vi "Reinitial Parameter After Test.vi"(8 "error in (no error)":errorcluster, 11 "main ref":T1) -> (0 "error out":errorcluster)   [LabVIEW 2025]
uses:
  controls/LAB-IQ UI Data.ctl
  Traction Loop/Traction Receipe Enum.ctl
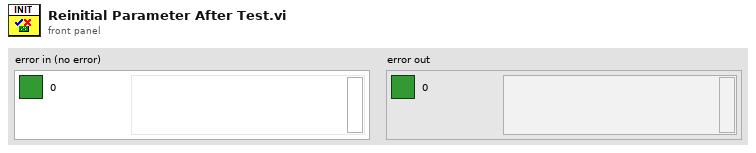
[diagram p1: front panel]
types:
  T1 = typedef "LAB-IQ UI Data.ctl" = cluster{"Main Home Screen":cluster{"GUI":refnum<vi>, "Platform Settings":refnum<vi>, "Configure":refnum<vi>, "Home":refnum<vi>, "EXIT":refnum<vi>, "service 2":refnum<vi>, "MainPage":refnum<vi>, "Analysis":refnum<vi>}, "Platform Settings":cluster{"mm/s  Surge":refnum<vi>, "Update Surge Speed":refnum<vi>, "Drive Error":refnum<vi>, "Disable Axis Jog Soft Limits":refnum<vi>, "mm/s  Sway":refnum<vi>, "Sway and Surge COM Status":refnum<vi>, "Heave COM Status":refnum<vi>, "Enable Platform":refnum<vi>, "Surge Forward Main":refnum<vi>, "Sway Right Main":refnum<vi>, "Sway Left Main":refnum<vi>, "Heave Down Main":refnum<vi>, "Heave Up main":refnum<vi>, "Update Sway Speed":refnum<vi>, "Update Heave Speed":refnum<vi>, "mm/s Heave":refnum<vi>, "mm/sec":refnum<vi>, "mm":refnum<vi>, "Surge Backward Main":refnum<vi>}, "Analysis Screen":cluster{"Analysis Home":refnum<vi>, "Surface Analysis":refnum<vi>, "Imaging":refnum<vi>, "Image Analysis":refnum<vi>, "Post Analysis":refnum<vi>}, "Config Screen":cluster{"Select Load Head":refnum<vi>, "Notes :":refnum<vi>, "FILE":refnum<vi>, "Sample ID :":refnum<vi>, "Operator ID :":refnum<vi>, "Operator Name :":refnum<vi>, "Auto":refnum<vi>}, "Motion Module":cluster{"zNL":refnum<vi>, "NL disp":refnum<vi>, "Rotary Tab":refnum<vi>, "Motion Direction:  3":refnum<vi>, "E.Velocity 2":refnum<vi>, "e.v/ssr 2":refnum<vi>, "Enter Fixed E.Velocity 2":refnum<vi>, "Enter Final SRR 2":refnum<vi>, "Enter initial SRR 2":refnum<vi>, "Enter Fixed SRR 2":refnum<vi>, "Enter the Final E.Velocity (m/s) 2":refnum<vi>, "Enter initial E.Velocity (m/s) 2":refnum<vi>, "Final Speed (RPM) 3":refnum<vi>, "Initial Speed (RPM) 2":refnum<vi>, "Enter the Final Velocity (m/s) 3":refnum<vi>, "Enter initial Velocity (m/s)  3":refnum<vi>, "Ramp Up 2":refnum<vi>, "TEST SELECTION":refnum<vi>, "SPEED SELECTION : ":refnum<vi>, "Angular Oscillation Set":refnum<vi>, "Traction":refnum<vi>, "Step Speed":refnum<vi>, "StepTable For Load-Speed":refnum<vi>, "StepTable For Speed":refnum<vi>, "Surge Forward MM":refnum<vi>, "Surge Backward MM":refnum<vi>, "M3 Image":refnum<vi>, "String 39":refnum<vi>, "Sway Left MM":refnum<vi>, "Sway Right MM":refnum<vi>, "Disable Axis Jog Soft Limits":refnum<vi>, "mm":refnum<vi>, "Heave Down MM":refnum<vi>, "Heave Up MM":refnum<vi>, "Wear Track Diameter (mm)":refnum<vi>, "Set WTD":refnum<vi>, "HomeScratch":refnum<vi>, "HomeRot":refnum<vi>, "PlaceModule":refnum<vi>, "Enter the Angle (Deg)":refnum<vi>, "Enter the Frequency (Hz)":refnum<vi>, "Motion Mode:":refnum<vi>, "LR Sway":refnum<vi>, "Rot Hor":refnum<vi>, "Scratch":refnum<vi>, "LR Cam":refnum<vi>, "MMBack":refnum<vi>, "MMNext":refnum<vi>, "Rot Ver":refnum<vi>, "Rotary Module Selection":refnum<vi>, "calculate rotary":refnum<vi>, "SPEED SELECTION : rotary":refnum<vi>, "Import 2":refnum<vi>, "Save 2":refnum<vi>, "File Path :  2":refnum<vi>, "String 45":refnum<vi>, "StepTable For Speed 3":refnum<vi>, "Enter the Speed(mm/sec)":refnum<vi>, "Enter the Speed(RPM)":refnum<vi>, "Enter Scratch Speed (mm/s):":refnum<vi>, "SwaySpeed Set":refnum<vi>, "Scartch Offset":refnum<vi>, "Motion type:":refnum<vi>, "HomeScratch 2":refnum<vi>, "Enter Scratch length (mm):":refnum<vi>, "Wear Track Diameter":refnum<vi>, "Rotary Speed Exced":refnum<vi>, "Scratch Mode":refnum<vi>, "No of Scratch":refnum<vi>}, "Environmental control":cluster{"Humidity  Status  3":refnum<vi>, "Low Temp  Status  2":refnum<vi>, "TK4 status 2":refnum<vi>, "Stage Temperature":refnum<vi>, "Sample Temperature":refnum<vi>, "Humidity (Amb)":refnum<vi>, "Clear List":refnum<vi>, "Add to list":refnum<vi>, "Wear":refnum<vi>, "Vibration":refnum<vi>, "Humidity (Chamber)":refnum<vi>, "Temperature (Chamber)":refnum<vi>, "ECR ":refnum<vi>, "Temperature (Amb)":refnum<vi>, "Microphone":refnum<vi>, "Acoustic Emission 3":refnum<vi>, "SNext":refnum<vi>, "APBack":refnum<vi>, "Enter the Temperature (°C):":refnum<vi>, "Enter the Stage \nTemperature (°C):":refnum<vi>, "Enter the Humidity (%Rh):":refnum<vi>, "Low Temp":refnum<vi>, "High Temp":refnum<vi>, "Humidity":refnum<vi>, "Sensors Picked":refnum<vi>}, "About Screen":cluster{"Password":refnum<vi>, "Home Service":refnum<vi>, "Advanced Setting":refnum<vi>, "About Tab":refnum<vi>, "ECR Port:":refnum<vi>, "Ramp Port:":refnum<vi>, "Installation/Replacement completed":refnum<vi>, "Loahead":refnum<vi>, "Heave and Surge COM Port:":refnum<vi>, "Sway COM Port:":refnum<vi>, "Temp Modbus:":refnum<vi>, "Humidity Port:":refnum<vi>, "Edit Gain Constants":refnum<vi>, "Save Gain Constants":refnum<vi>}, "Main Screen":cluster{"Main Screen Tab":refnum<vi>, "Angle and Frequency":refnum<vi>, "Stroke (mm)":refnum<vi>, "Angle (Deg)":refnum<vi>, "Main Speed Tab":refnum<vi>, "MTM MOTOR DISPLAY":refnum<vi>, "Disc Speed (m/sec)":refnum<vi>, "Ball Speed (m/sec)":refnum<vi>, "Disc Speed (RPM)":refnum<vi>, "Ball Speed (RPM)":refnum<vi>, "SPEED TAB":refnum<vi>, "Speed (m/sec)":refnum<vi>, "Set Speed (m/sec)":refnum<vi>, "Speed (RPM)":refnum<vi>, "Set Speed":refnum<vi>, "Time Tab":refnum<vi>, "Time ( HH:MM:SS ) 2":refnum<vi>, "Test Duration":refnum<vi>, "Test Duration 4":refnum<vi>, "TEST CYCLE":refnum<vi>, "TOTAL CYCLES":refnum<vi>, "Set Load (N)":refnum<vi>, "Temp Tabs":refnum<vi>, "Heater":refnum<vi>, "TK4 status":refnum<vi>, "ChamberTemp":refnum<vi>, "SetTmp":refnum<vi>, "Controller  Status":refnum<vi>, "ChamberTemp 2":refnum<vi>, "SetTmp 2":refnum<vi>, "Controller  Status 2":refnum<vi>, "ChamberTemp 3":refnum<vi>, "SetTmp 3":refnum<vi>, "Cooling":refnum<vi>, "Load Communication":refnum<vi>, "Ambient \nTemperature":refnum<vi>, "HumCOMStatus":refnum<vi>, "Ambient\n Humidity":refnum<vi>, "Freq (Hz)":refnum<vi>, "Load En":refnum<vi>, "NLt":refnum<vi>, "zNL 2":refnum<vi>, "Humidity On":refnum<vi>, "humidity disp":refnum<vi>, "Set Humidity":refnum<vi>, "NL disp 2":refnum<vi>, "Humidity On 2":refnum<vi>, "humidity disp 2":refnum<vi>, "Set Humidity 2":refnum<vi>, "NL disp 3":refnum<vi>, "AppLoadSeq scratch":refnum<vi>, "Stop Scratch":refnum<vi>, "ClrLog":refnum<vi>, "Trip Log":refnum<vi>, "STOP":refnum<vi>, "Start Test":refnum<vi>, "Test status":refnum<vi>, "AR Led":refnum<vi>, "Data":refnum<vi>, "Health":refnum<vi>, "Sway COM Status":refnum<vi>, "Heave COM Status":refnum<vi>, "Grp Tab":refnum<vi>, "Sub Graph":refnum<vi>, "SD (mm)":refnum<vi>, "Siliding distance Reset Graph":refnum<vi>, "SDGp":refnum<vi>, "Humidity Reset Graph":refnum<vi>, "HumrGp":refnum<vi>, "Acoustic Emission (mV)":refnum<vi>, "Aqucostic Reset Graph":refnum<vi>, "gACQUOS":refnum<vi>, "ECR RESET":refnum<vi>, "ECR":refnum<vi>, "Temperature Reset":refnum<vi>, "Acoustic Emission (mV) 2":refnum<vi>, "Aqucostic Reset Graph 2":refnum<vi>, "gACQUOS 2":refnum<vi>, "ECR RESET 2":refnum<vi>, "ECR 2":refnum<vi>, "Temperature Reset 2":refnum<vi>, "Temperature (deg c)":refnum<vi>, "Speed Reset Graph":refnum<vi>, "Speed Tab":refnum<vi>, "MTM DISC  SPEED":refnum<vi>, "MTM BALL SPEED":refnum<vi>, "speed mm/sec":refnum<vi>, "Hymidity":refnum<vi>, "Humidity Disable trip":refnum<vi>, "CoF Trip  2":refnum<vi>, "Depth Trip":refnum<vi>, "Weart Deapth":refnum<vi>, "Depth Reset Graph":refnum<vi>, "Weart":refnum<vi>, "Depthz":refnum<vi>, "Depth (µm)":refnum<vi>, "WearGp":refnum<vi>, "NL Trip 2":refnum<vi>, "Load pid":refnum<vi>, "Load Disable Trip":refnum<vi>, "Load Reset Graph":refnum<vi>, "NL Display 4":refnum<vi>, "Main Chart 3":refnum<vi>, "BACK":refnum<vi>, "Depth Trip 2":refnum<vi>, "COF TRIP ":refnum<vi>, "Friction Force (N)":refnum<vi>, "FF Reset Graph":refnum<vi>, "FF Disable Trip":refnum<vi>, "FF TRIP":refnum<vi>, "COF Disable Trip":refnum<vi>, "COF Reset Graph":refnum<vi>, "Start Test Temp":refnum<vi>, "zFF":refnum<vi>, "Friction Force (N) Graph":refnum<vi>, "Coefficient of Friction":refnum<vi>, "Scratch Start Test":refnum<vi>, "FF Tab":refnum<vi>, "Cyclic Friction Force (N)":refnum<vi>, "CZ FF":refnum<vi>, "Cyclic Friction Force (N) Graph":refnum<vi>, "Cyclic Coefficient of Friction":refnum<vi>, "Cyclic FF TRIP":refnum<vi>, "Cyclic FF Disable Trip":refnum<vi>, "cyclic COF Disable Trip":refnum<vi>, "cyclic COF TRIP":refnum<vi>, "cyclic COF Reset Graph":refnum<vi>, "Cyclic FF Reset Graph":refnum<vi>, "Test Trip":refnum<vi>, "Multi Scratch Pass":refnum<vi>, "Scratch Start Recording":refnum<vi>}, "Loading":cluster{"Indentation":refnum<vi>, "Reference Sample":refnum<vi>, "Load Cell Communication Slide":refnum<vi>, "com 3":refnum<vi>, "com":refnum<vi>, "DecaForce COM Status":refnum<vi>, "Update":refnum<vi>, "Clear 3":refnum<vi>, "seq":refnum<vi>, "Stribeck table":refnum<vi>, "Stribeck Table  For loading":refnum<vi>, "Loading Mode":refnum<vi>, "Enter the Final Load (N)":refnum<vi>, "Enter the CoF Trip":refnum<vi>, "Enter the Friction Force Trip":refnum<vi>, "Enter the Normal load Trip":refnum<vi>, "Enter the Load  (N)":refnum<vi>, "KiloForce":refnum<vi>, "DecaForce ":refnum<vi>, "MicroForce":refnum<vi>, "LHBack":refnum<vi>, "LHNext":refnum<vi>, "Enter the Loading Rate (N/min)":refnum<vi>, "Message":refnum<vi>, "Warning 2":refnum<vi>, "SSP 0.75":refnum<vi>, "SSP 0.5":refnum<vi>, "SSP 0.3":refnum<vi>, "Warning":refnum<vi>, "gui GIF":refnum<vi>, "Communication is established":refnum<vi>, "AppLoad 4":refnum<vi>, "Multipoint":refnum<vi>, "Load Selection":refnum<vi>}, "PID":cluster{"Ramp MulFac":refnum<vi>, "pulses LoadDiffRamp(2..10)":refnum<vi>, "PulseControlRamp(diff<=3N)":refnum<vi>, "SetLoadDeadband(%) Load(0-10N)":refnum<vi>, "PID gains out delay (microForce)":refnum<vi>, "Ramp":refnum<vi>, "Gain 2":refnum<vi>, "pulses LoadDiff(2..10)":refnum<vi>, "pulses LoadDiff(11..50)":refnum<vi>, "PulseControl(diff<=3N)":refnum<vi>, "SetLoadDeadband(%)  2":refnum<vi>, "Dummy Run":refnum<vi>, "Vertical load (N)":refnum<vi>, "AutoTune":refnum<vi>, "Offset 3 ":refnum<vi>, "apply load":refnum<vi>, "Offset  3":refnum<vi>, "apply load 2":refnum<vi>, "Enter ByPass Load":refnum<vi>, "reinit 3":refnum<vi>, "output range delay":refnum<vi>, "PID gains out delay":refnum<vi>, "Bypass Load":refnum<vi>, "pulsesSent":refnum<vi>, "pulses ":refnum<vi>, "actpid":refnum<vi>, "gFF Rot":refnum<vi>, "pulses LoadDiff(21..1000)":refnum<vi>, "Delay":refnum<vi>, "deadband":refnum<vi>}, "Config Parameters":cluster{"Tab Control 3":refnum<vi>, "Tab Control 19":refnum<vi>, "SAMPLES":refnum<vi>, "Re-initilaize":refnum<vi>, "Filter ON/OFF":refnum<vi>, "TracHomeSurgeOffsetCounts 10MM":refnum<vi>, "TracHomeSwayOffsetCounts 10MM":refnum<vi>, "Acoustic Emission:":refnum<vi>, "Apply Filter (FF)":refnum<vi>, "Filter% 2":refnum<vi>, "Apply Filter (Load)":refnum<vi>, "Filter% ":refnum<vi>, "Sway distance (mm)":refnum<vi>, "Surge distance (mm)":refnum<vi>, "DataSavingLoopDelay(ms)":refnum<vi>, "SAVE 2":refnum<vi>, "Enter Distance":refnum<vi>, "Sway Counts:":refnum<vi>, "Distance (mm): 3":refnum<vi>, "Surge Counts:":refnum<vi>, "Distance (mm): 2":refnum<vi>, "Distance (mm):":refnum<vi>, "Heave Counts:":refnum<vi>, "LRMHomeSurgeOffsetCounts":refnum<vi>, "LRMHomeSwayOffsetCounts":refnum<vi>, "TracHomeSurgeOffsetCounts 20MM":refnum<vi>, "TracHomeSwayOffsetCounts 20MM":refnum<vi>, "RotHomeSwayOffsetCounts":refnum<vi>, "RotHomeSurgeOffsetCounts":refnum<vi>, "Heave distance":refnum<vi>, "Zmm":refnum<vi>, "Heave Pulses/mm":refnum<vi>, "Surge Pulses/mm":refnum<vi>, "Sway Pulses/mm":refnum<vi>, "Heave Pitch":refnum<vi>, "Surge Pitch":refnum<vi>, "Sway Pitch":refnum<vi>, "Heave PPR":refnum<vi>, "Surge PPR":refnum<vi>, "Sway PPR":refnum<vi>, "Tab Control 5":refnum<vi>, "Tab Control 14":refnum<vi>, "Tab Control 26":refnum<vi>, "AE":refnum<vi>, "Heave Loop Delay":refnum<vi>, "Heave PID Speed":refnum<vi>, "Surge Jog Speed":refnum<vi>, "Heave Jog Speed":refnum<vi>, "Sway Loop Delay":refnum<vi>, "Sway PID Speed":refnum<vi>, "Sway Jog Speed":refnum<vi>, "DEPTH TRIP VALUE":refnum<vi>, "LOAD TRIP VALUE":refnum<vi>, "DEPTH TRIP   ENABLE":refnum<vi>, "LOAD TRIP  ENABLE":refnum<vi>, "CYCLIC FF TRIP VALUE":refnum<vi>, "FF TRIP VALUE":refnum<vi>, "CYCLIC CoF TRIP VALUE":refnum<vi>, "COF TRIP VALUE":refnum<vi>, "CYCLIC COF TRIP  ENABLE":refnum<vi>, "CYCLIC FF TRIP  ENABLE":refnum<vi>, "FF TRIP  ENABLE":refnum<vi>, "COF TRIP  ENABLE":refnum<vi>, "JOG TRIP LOAD VALUE (N)":refnum<vi>}, "Loading Com Port":cluster{"ClearAll":refnum<vi>, "Mz(Nm)":refnum<vi>, "My(Nm)":refnum<vi>, "Mx(Nm)":refnum<vi>, "Save Dwell":refnum<vi>, "Mx ":refnum<vi>, "My ":refnum<vi>, "Mz":refnum<vi>, "Fx(N)":refnum<vi>, "Fy(N)":refnum<vi>, "Fz(N)":refnum<vi>, "ZeroAll":refnum<vi>, "Acq Delay (ms)":refnum<vi>, "Burst Delay (ms)":refnum<vi>, "model":refnum<vi>, "SN":refnum<vi>, "FFx(N)":refnum<vi>, "Sensor IP":refnum<vi>, "Port":refnum<vi>, "FFy(N)":refnum<vi>, "Load(N)":refnum<vi>, "delete Handle":refnum<vi>, "Create Handle":refnum<vi>, "ft_data":refnum<vi>, "ft_range":refnum<vi>, "ft_data 2":refnum<vi>, "stop 6":refnum<vi>, "running_flag":refnum<vi>, "ft_udp_handle":refnum<vi>, "get-data-return":refnum<vi>, "get-range-return":refnum<vi>, "zero-return":refnum<vi>, "filter-return":refnum<vi>, "initial-return":refnum<vi>, "deleteHandle-result":refnum<vi>, "Load Cell Temp":refnum<vi>}, "Heave AND Surge":cluster{"SURGE POSE":refnum<vi>, "error out Read":refnum<vi>, "HEAVE POSE":refnum<vi>, "State":refnum<vi>, "Homed":refnum<vi>, "Sequence ID":refnum<vi>, "error out Write":refnum<vi>, "faultCode":refnum<vi>, "Ack ID":refnum<vi>, "SPEED":refnum<vi>, "Distance":refnum<vi>, "Mode Command":refnum<vi>, "Heave and Surge Read":refnum<vi>, "Read Heave Temp":refnum<vi>, "Spare 15":refnum<vi>, "Spare 14":refnum<vi>, "Spare 13":refnum<vi>, "Spare 12":refnum<vi>, "Spare 11":refnum<vi>, "Spare 10":refnum<vi>, "Spare 9":refnum<vi>, "Spare 8":refnum<vi>, "Spare 7":refnum<vi>, "Spare 6":refnum<vi>, "Spare 5":refnum<vi>, "Spare 4":refnum<vi>, "Spare 2":refnum<vi>, "Spare 1":refnum<vi>, "Node Id":refnum<vi>, "Spare 3":refnum<vi>, "SPARE 4":refnum<vi>, "SPARE 3":refnum<vi>, "SPARE 2":refnum<vi>, "SPARE 1":refnum<vi>, "fwMajor":refnum<vi>, "fwMinor":refnum<vi>, "Manual Write":refnum<vi>, "Heave and Surge Write":refnum<vi>, "SPARE 5":refnum<vi>, "Reserved ":refnum<vi>, "SPARE 8":refnum<vi>, "SPARE 6":refnum<vi>, "SPARE 7":refnum<vi>, "SPARE 17":refnum<vi>, "SPARE 16":refnum<vi>, "SPARE 15":refnum<vi>, "SPARE 14":refnum<vi>, "SPARE 13":refnum<vi>, "SPARE 12":refnum<vi>, "SPARE 11":refnum<vi>, "SPARE 10":refnum<vi>, "SPARE 9":refnum<vi>, "System UPTIME":refnum<vi>, "Missed Packets":refnum<vi>, "faultCode Surge Right":refnum<vi>, "faultCode Surge Left":refnum<vi>, "faultCode Heave":refnum<vi>, "UPLINK HEAVE":refnum<vi>, "DOWNLINK HEAVE":refnum<vi>}, "New PID LOGIC":cluster{"Fine Tune Zone":refnum<vi>, "PID SDelay":refnum<vi>, "Max_pos_limit":refnum<vi>, "Min_pos_limit":refnum<vi>, "i_limit":refnum<vi>, "pct_scale":refnum<vi>, "Deadband":refnum<vi>, "Kd":refnum<vi>, "Ki":refnum<vi>, "Kp":refnum<vi>, "Current Position":refnum<vi>, "Set Load":refnum<vi>, "Current Load":refnum<vi>, "Pulse delta":refnum<vi>, "Init Step":refnum<vi>, "Max Step Linit":refnum<vi>, "min_deadband_floor":refnum<vi>, "dynamic_spindle_noise_scalar":refnum<vi>, "min_finetune_floor":refnum<vi>, "filter_alpha":refnum<vi>}, "SWAY ":cluster{"fwMajor":refnum<vi>, "Homed":refnum<vi>, "Rotary POSE":refnum<vi>, "State":refnum<vi>, "SWAY POSE":refnum<vi>, "Ack ID":refnum<vi>, "faultCode":refnum<vi>, "Node Id":refnum<vi>, "fwMinor":refnum<vi>, "Spare 6":refnum<vi>, "Spare 5":refnum<vi>, "Spare 4":refnum<vi>, "Spare 3":refnum<vi>, "Spare 2":refnum<vi>, "Spare 1":refnum<vi>, "Spare 7":refnum<vi>, "SPARE  5":refnum<vi>, "error out Write  SWAY ":refnum<vi>, "error out Read SWAY ":refnum<vi>, "Manual Write SWAY ":refnum<vi>, "SWAY WRITE":refnum<vi>, "SPARE  4":refnum<vi>, "SPARE  3":refnum<vi>, "SPARE 2":refnum<vi>, "SPARE 1":refnum<vi>, "Spare 15":refnum<vi>, "Spare 14":refnum<vi>, "Spare 13":refnum<vi>, "Spare 12":refnum<vi>, "Spare 11":refnum<vi>, "Spare 9":refnum<vi>, "Spare 8":refnum<vi>, "SPEED":refnum<vi>, "Distance":refnum<vi>, "Mode Command":refnum<vi>, "Sequence ID":refnum<vi>, "SWAY READ":refnum<vi>, "Spare 10":refnum<vi>, "Read SWAY Temp":refnum<vi>, "faultCode Sway ":refnum<vi>, "Missed Packets":refnum<vi>, "System UPTIME sway":refnum<vi>, "SPARE 6":refnum<vi>, "SPARE 7":refnum<vi>, "SPARE 9":refnum<vi>, "SPARE 11":refnum<vi>, "SPARE 10":refnum<vi>, "SPARE 8":refnum<vi>, "SPARE 13":refnum<vi>, "SPARE 12":refnum<vi>, "SPARE 17":refnum<vi>, "SPARE 16":refnum<vi>, "SPARE 15":refnum<vi>, "SPARE 14":refnum<vi>, "Reserved":refnum<vi>, "faultCode Rotary":refnum<vi>, "UPLINK SWAY":refnum<vi>, "DOWNLINK SWAY":refnum<vi>}, "Analysis Screen":cluster{"Analysis Home":refnum<vi>, "Refresh 2":refnum<vi>, "MEAN 4":refnum<vi>, "SD 4":refnum<vi>, "VARIANCE 4":refnum<vi>, "MEAN  3":refnum<vi>, "SD  3":refnum<vi>, "VARIANCE  3":refnum<vi>, "MEAN 2":refnum<vi>, "SD  2":refnum<vi>, "VARIANCE 2":refnum<vi>, "MEAN":refnum<vi>, "SD":refnum<vi>, "VARIANCE":refnum<vi>, "File 4 Discription":refnum<vi>, "OPEN 4":refnum<vi>, "File Name 4":refnum<vi>, "OPEN 3":refnum<vi>, "File 3 Discription":refnum<vi>, "File Name 3":refnum<vi>, "Y-AXIS":refnum<vi>, "X-AXIS":refnum<vi>, "XY Graph":refnum<vi>, "File Name 2":refnum<vi>, "File Name 1":refnum<vi>, "OPEN 2":refnum<vi>, "OPEN 1":refnum<vi>, "File 1 Discription ":refnum<vi>, "File 2 Discription":refnum<vi>, "Export":refnum<vi>, "File Format":refnum<vi>}, "Traction":cluster{"faultCode Traction 2":refnum<vi>, "faultCode Traction 1":refnum<vi>, "Missed Packets":refnum<vi>, "System UPTIME Traction":refnum<vi>, "SPARE 17":refnum<vi>, "SPARE 16":refnum<vi>, "SPARE 15":refnum<vi>, "SPARE 14":refnum<vi>, "SPARE 13":refnum<vi>, "SPARE 12":refnum<vi>, "SPARE 11":refnum<vi>, "SPARE 10":refnum<vi>, "SPARE 9":refnum<vi>, "SPARE 8":refnum<vi>, "SPARE 7":refnum<vi>, "SPARE 6":refnum<vi>, "Reserved":refnum<vi>, "SPARE  5":refnum<vi>, "Manual Write TRACTION":refnum<vi>, "TRACTION WRITE":refnum<vi>, "SPARE  4":refnum<vi>, "SPARE  3":refnum<vi>, "SPARE 2":refnum<vi>, "SPARE 1":refnum<vi>, "Spare 7":refnum<vi>, "Spare 6":refnum<vi>, "Spare 5":refnum<vi>, "Spare 4":refnum<vi>, "Spare 2":refnum<vi>, "Spare 1":refnum<vi>, "Node Id":refnum<vi>, "Read TRACTION Temp":refnum<vi>, "fwMinor":refnum<vi>, "fwMajor":refnum<vi>, "faultCode":refnum<vi>, "TRACTION POSE":refnum<vi>, "TRACTION POSE 2":refnum<vi>, "Homed":refnum<vi>, "State":refnum<vi>, "Ack ID":refnum<vi>, "SPEED":refnum<vi>, "Distance":refnum<vi>, "Mode Command":refnum<vi>, "Sequence ID":refnum<vi>, "error out Read TRACTION":refnum<vi>, "error out Write  TRACTION":refnum<vi>, "TRACTION READ":refnum<vi>, "Spare 3":refnum<vi>}, "Traction reciepe":cluster{"SRR Sweep Range (%) Stribeck":refnum<vi>, "Traction Receipe":refnum<vi>, "Total Execution Time":refnum<vi>, "Total Steps":refnum<vi>, "Duration / Step (s)  Stribeck":refnum<vi>, "STRIBECK Fixed SRR List (%)":refnum<vi>, "Duration / Step (s) Traction":refnum<vi>, "SRR Sweep Range (%) traction":refnum<vi>, "Rolling Speed (mm/s)":refnum<vi>, "Temperature Stages (°C)":refnum<vi>, "Ball Load (N)":refnum<vi>, "Lubricant Name":refnum<vi>, "Profile File Name":refnum<vi>, "SET entrainment Velocity":refnum<vi>, "Test Array Size":refnum<vi>, "SRR INDEX [ STRIBECK]":refnum<vi>, "Stribeck Size":refnum<vi>, "SET SRR":refnum<vi>, "ELAPSED TIMER ":refnum<vi>, "BALL SET RPM":refnum<vi>, "DISC SET RPM":refnum<vi>, "SET LOAD":refnum<vi>, "TEMPERATURE READ":refnum<vi>, "SET TEMPERATURE":refnum<vi>, "Traction Size":refnum<vi>, "DISC SPEED (rpm)":refnum<vi>, "BALL SPEED (rpm)":refnum<vi>, "BALL WEAR TRACK":refnum<vi>, "DISC WEARTRACK":refnum<vi>, "SRR INDEX [ TRACTION]":refnum<vi>, "Start Index Type":refnum<vi>, "Enum - Menu":refnum<vi>, "Ball (mm/sec)":refnum<vi>, "Disc (mm/sec)":refnum<vi>}, "Traction Control":cluster{"HomeTraction":refnum<vi>, "Demo Mode Display":refnum<vi>, "Traction Message":refnum<vi>, "Traction Step Update Details":refnum<vi>, "Main Tab sequence for selection":refnum<vi>, "Ramp Tab":refnum<vi>, "e.v/ssr":refnum<vi>, "Enter Fixed E.Velocity":refnum<vi>, "Enter Final SRR":refnum<vi>, "Enter initial SRR":refnum<vi>, "Enter Fixed SRR":refnum<vi>, "Enter the Final E.Velocity (m/s)":refnum<vi>, "Enter initial E.Velocity (m/s)":refnum<vi>, "Ball WTD":refnum<vi>, "E.Velocity":refnum<vi>, "Enter the Final Velocity (m/s)":refnum<vi>, "Enter initial Velocity (m/s)":refnum<vi>, "Ramp Up   Disc":refnum<vi>, "Initial DiscSpeed (RPM)":refnum<vi>, "Final Speed (RPM) Ball":refnum<vi>, "Final Speed (RPM)":refnum<vi>, "Initial Speed (RPM) Ball":refnum<vi>, "Enter the Final Velocity (m/s) Ball":refnum<vi>, "Enter initial Velocity (m/s) Ball":refnum<vi>, "Ramp Up":refnum<vi>, "ExceedBallSpeed step":refnum<vi>, "ExceedDiscSpeed":refnum<vi>, "BallSpeed Exceed Indication":refnum<vi>, "Apply":refnum<vi>, "SPEED SELECTION : MTM":refnum<vi>, "SPEED SELECTION : MTM 2":refnum<vi>, "TEST SELECTION (MTM)":refnum<vi>, "MTM Test Selection":refnum<vi>, "File Path Tab":refnum<vi>, "File Path String":refnum<vi>, "Save":refnum<vi>, "Save  2":refnum<vi>, "Import ":refnum<vi>, "File Path :":refnum<vi>, "Step Sequence Indication Tab":refnum<vi>, "Step Sequence Indication":refnum<vi>, "Calculate Step":refnum<vi>, "StepTable":refnum<vi>, "ExceedDiscSpeed  Cinstant Speed":refnum<vi>, "ExceedBallSpeed Constant":refnum<vi>, "TEST SELECTION (MTM) 2":refnum<vi>, "SPEED SELECTION : MTM 3":refnum<vi>, "MTM Test Selection 2":refnum<vi>, "Enter the Speed (m/sec): ":refnum<vi>, "Enter the Speed (m/sec):  2":refnum<vi>, "Enter the Speed (RPM):":refnum<vi>, "Lower Spped ":refnum<vi>, "Upper":refnum<vi>, "Enter the Speed (RPM):Ball":refnum<vi>, "Disc Motion Direction: ":refnum<vi>, "Ball Motion Direction :":refnum<vi>, "Motion Mode: ":refnum<vi>, "Wear Track Diameter (mm) ":refnum<vi>, "Disc Speed Indicator":refnum<vi>, "ExceedBallSpeed":refnum<vi>}, "Acquostic":cluster{"Last Config Rejected ":refnum<vi>, "rx command count":refnum<vi>, "Current Filter Id":refnum<vi>, "Isolated Gain":refnum<vi>, "DAQ Status":refnum<vi>, "error out":refnum<vi>, "error in (no error)":refnum<vi>, "Uplink Packet":refnum<vi>, "data out":refnum<vi>, "Downlink Packet":refnum<vi>, "Signal Energy":refnum<vi>, "Amplitude db_AE":refnum<vi>, "Peak Amplitude":refnum<vi>, "AE Ring-Down Counts":refnum<vi>, "Gains":refnum<vi>, "Manual Write Acquostic":refnum<vi>}}
  T2 = enum8{"Enabled", "Disabled", "Disabled and Grayed Out"}
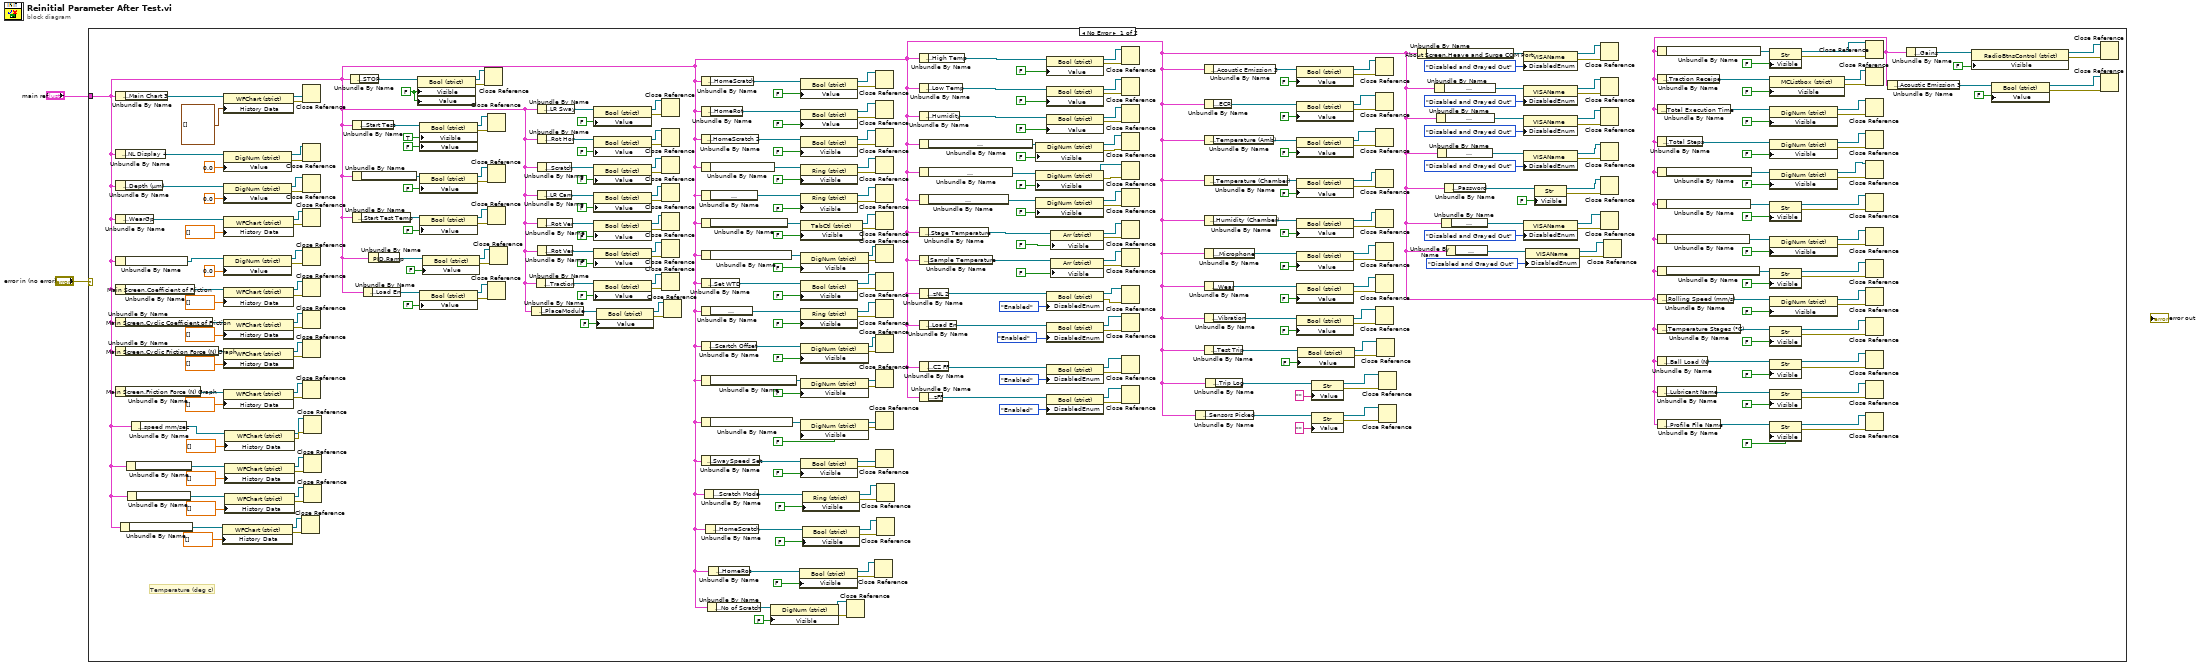
[diagram p0: block diagram]
diagram:
  n1 = case shown="No Error" "error in (no error)" {
    tunnel: "main ref" -> [w4 _]
    frame No Error {
      w293 = FALSE ("Visible")
      # "Temperature (deg c)"
      n2 = Unbundle By Name(w4) -> ("Main Screen.Main Chart 3"=w358:refnum<vi>)
      n3 = Unbundle By Name(w4) -> ("Main Screen.NL Display 4"=w356:refnum<vi>)
      n4 = Unbundle By Name(w4) -> ("Main Screen.Depth (µm)"=w351:refnum<vi>)
      n5 = Unbundle By Name(w4) -> ("Main Screen.WearGp"=w348:refnum<vi>)
      n6 = Unbundle By Name(w4) -> ("Main Screen.Time ( HH:MM:SS ) 2"=w344:refnum<vi>)
      n7 = Unbundle By Name(w4) -> ("Main Screen.Coefficient of Friction"=w341:refnum<vi>)
      n8 = Unbundle By Name(w4) -> ("Main Screen.Cyclic Coefficient of Friction"=w333:refnum<vi>)
      n9 = Unbundle By Name(w4) -> ("Main Screen.Cyclic Friction Force (N) Graph"=w337:refnum<vi>)
      n10 = Unbundle By Name(w4) -> ("Main Screen.Friction Force (N) Graph"=w329:refnum<vi>)
      n11 = Unbundle By Name(w4) -> ("Main Screen.Temperature (deg c)"=w312:refnum<vi>)
      n12 = Unbundle By Name(w4) -> ("Main Screen.MTM DISC  SPEED"=w319:refnum<vi>)
      n13 = Unbundle By Name(w4) -> ("Main Screen.MTM BALL SPEED"=w314:refnum<vi>)
      n14 = Unbundle By Name(w4) -> ("Main Screen.speed mm/sec"=w322:refnum<vi>)
      n15 = property class="WFChart (strict)"(reference=w312, "History Data"=dbl[] []) -> (reference out=w309:refnum<vi>, error out=w311:errorcluster)  [unwired: 1 in]
      n16 = property class="WFChart (strict)"(reference=w358, "History Data"=cluster{dbl, "NL disp":dbl, dbl}[] []) -> (reference out=w360:refnum<vi>, error out=w359:errorcluster)  [unwired: 1 in]
      n17 = property class="DigNum (strict)"(reference=w356, "Value"=0.0) -> (reference out=w354:refnum<vi>, error out=w355:errorcluster)  [unwired: 1 in]
      n18 = property class="DigNum (strict)"(reference=w351, "Value"=0.0) -> (reference out=w352:refnum<vi>, error out=w350:errorcluster)  [unwired: 1 in]
      n19 = property class="WFChart (strict)"(reference=w348, "History Data"=dbl[] []) -> (reference out=w346:refnum<vi>, error out=w347:errorcluster)  [unwired: 1 in]
      n20 = property class="DigNum (strict)"(reference=w344, "Value"=0.0) -> (reference out=w325:refnum<vi>, error out=w345:errorcluster)  [unwired: 1 in]
      n21 = property class="WFChart (strict)"(reference=w341, "History Data"=dbl[] []) -> (reference out=w342:refnum<vi>, error out=w340:errorcluster)  [unwired: 1 in]
      n22 = property class="WFChart (strict)"(reference=w333, "History Data"=dbl[] []) -> (reference out=w332:refnum<vi>, error out=w334:errorcluster)  [unwired: 1 in]
      n23 = property class="WFChart (strict)"(reference=w337, "History Data"=dbl[] []) -> (reference out=w335:refnum<vi>, error out=w336:errorcluster)  [unwired: 1 in]
      n24 = property class="WFChart (strict)"(reference=w329, "History Data"=dbl[] []) -> (reference out=w327:refnum<vi>, error out=w328:errorcluster)  [unwired: 1 in]
      n25 = property class="WFChart (strict)"(reference=w322, "History Data"=dbl[] []) -> (reference out=w321:refnum<vi>, error out=w323:errorcluster)  [unwired: 1 in]
      n26 = property class="WFChart (strict)"(reference=w319, "History Data"=dbl[] []) -> (reference out=w320:refnum<vi>, error out=w318:errorcluster)  [unwired: 1 in]
      n27 = property class="WFChart (strict)"(reference=w314, "History Data"=dbl[] []) -> (reference out=w313:refnum<vi>, error out=w315:errorcluster)  [unwired: 1 in]
      n28 = Close Reference(reference=w309, error in (no error)=w311) -> ()  [unwired: 1 out]
      n29 = Close Reference(reference=w360, error in (no error)=w359) -> ()  [unwired: 1 out]
      n30 = Close Reference(reference=w354, error in (no error)=w355) -> ()  [unwired: 1 out]
      n31 = Close Reference(reference=w352, error in (no error)=w350) -> ()  [unwired: 1 out]
      n32 = Close Reference(reference=w346, error in (no error)=w347) -> ()  [unwired: 1 out]
      n33 = Close Reference(reference=w325, error in (no error)=w345) -> ()  [unwired: 1 out]
      n34 = Close Reference(reference=w342, error in (no error)=w340) -> ()  [unwired: 1 out]
      n35 = Close Reference(reference=w332, error in (no error)=w334) -> ()  [unwired: 1 out]
      n36 = Close Reference(reference=w335, error in (no error)=w336) -> ()  [unwired: 1 out]
      n37 = Close Reference(reference=w327, error in (no error)=w328) -> ()  [unwired: 1 out]
      n38 = Close Reference(reference=w321, error in (no error)=w323) -> ()  [unwired: 1 out]
      n39 = Close Reference(reference=w320, error in (no error)=w318) -> ()  [unwired: 1 out]
      n40 = Close Reference(reference=w313, error in (no error)=w315) -> ()  [unwired: 1 out]
      n41 = Unbundle By Name(w4) -> ("Main Screen.STOP"=w299:refnum<vi>)
      n42 = Unbundle By Name(w4) -> ("Main Screen.Start Test"=w297:refnum<vi>)
      n43 = Unbundle By Name(w4) -> ("Main Screen.Scratch Start Test"=w305:refnum<vi>)
      n44 = Unbundle By Name(w4) -> ("Main Screen.Start Test Temp"=w306:refnum<vi>)
      n45 = Unbundle By Name(w4) -> ("Main Screen.Load En"=w285:refnum<vi>)
      n46 = Unbundle By Name(w4) -> ("PID.Ramp"=w290:refnum<vi>)
      n47 = property class="Bool (strict)"(reference=w299, "Visible"=w293, "Value"=w293) -> (reference out=w294:refnum<vi>, error out=w300:errorcluster)  [unwired: 1 in]
      n48 = property class="Bool (strict)"(reference=w297, "Visible"=TRUE, "Value"=FALSE) -> (reference out=w295:refnum<vi>, error out=w296:errorcluster)  [unwired: 1 in]
      n49 = property class="Bool (strict)"(reference=w305, "Value"=FALSE) -> (reference out=w303:refnum<vi>, error out=w304:errorcluster)  [unwired: 1 in]
      n50 = property class="Bool (strict)"(reference=w306, "Value"=FALSE) -> (reference out=w308:refnum<vi>, error out=w307:errorcluster)  [unwired: 1 in]
      n51 = property class="Bool (strict)"(reference=w285, "Value"=FALSE) -> (reference out=w287:refnum<vi>, error out=w286:errorcluster)  [unwired: 1 in]
      n52 = property class="Bool (strict)"(reference=w290, "Value"=FALSE) -> (reference out=w288:refnum<vi>, error out=w289:errorcluster)  [unwired: 1 in]
      n53 = Close Reference(reference=w294, error in (no error)=w300) -> ()  [unwired: 1 out]
      n54 = Close Reference(reference=w295, error in (no error)=w296) -> ()  [unwired: 1 out]
      n55 = Close Reference(reference=w303, error in (no error)=w304) -> ()  [unwired: 1 out]
      n56 = Close Reference(reference=w308, error in (no error)=w307) -> ()  [unwired: 1 out]
      n57 = Close Reference(reference=w287, error in (no error)=w286) -> ()  [unwired: 1 out]
      n58 = Close Reference(reference=w288, error in (no error)=w289) -> ()  [unwired: 1 out]
      n59 = Unbundle By Name(w4) -> ("Motion Module.PlaceModule"=w254:refnum<vi>)
      n60 = Unbundle By Name(w4) -> ("Motion Module.Traction"=w258:refnum<vi>)
      n61 = Unbundle By Name(w4) -> ("Motion Module.LR Sway"=w281:refnum<vi>)
      n62 = Unbundle By Name(w4) -> ("Motion Module.Rot Hor"=w278:refnum<vi>)
      n63 = Unbundle By Name(w4) -> ("Motion Module.Scratch"=w274:refnum<vi>)
      n64 = Unbundle By Name(w4) -> ("Motion Module.LR Cam"=w269:refnum<vi>)
      n65 = Unbundle By Name(w4) -> ("Motion Module.Rot Ver"=w266:refnum<vi>)
      n66 = Unbundle By Name(w4) -> ("Motion Module.Rot Ver"=w262:refnum<vi>)
      n67 = property class="Bool (strict)"(reference=w281, "Value"=FALSE) -> (reference out=w283:refnum<vi>, error out=w282:errorcluster)  [unwired: 1 in]
      n68 = property class="Bool (strict)"(reference=w278, "Value"=FALSE) -> (reference out=w276:refnum<vi>, error out=w277:errorcluster)  [unwired: 1 in]
      n69 = property class="Bool (strict)"(reference=w274, "Value"=FALSE) -> (reference out=w272:refnum<vi>, error out=w275:errorcluster)  [unwired: 1 in]
      n70 = property class="Bool (strict)"(reference=w269, "Value"=FALSE) -> (reference out=w271:refnum<vi>, error out=w268:errorcluster)  [unwired: 1 in]
      n71 = property class="Bool (strict)"(reference=w266, "Value"=FALSE) -> (reference out=w264:refnum<vi>, error out=w267:errorcluster)  [unwired: 1 in]
      n72 = property class="Bool (strict)"(reference=w262, "Value"=FALSE) -> (reference out=w260:refnum<vi>, error out=w261:errorcluster)  [unwired: 1 in]
      n73 = property class="Bool (strict)"(reference=w258, "Value"=FALSE) -> (reference out=w256:refnum<vi>, error out=w257:errorcluster)  [unwired: 1 in]
      n74 = property class="Bool (strict)"(reference=w254, "Value"=FALSE) -> (reference out=w252:refnum<vi>, error out=w253:errorcluster)  [unwired: 1 in]
      n75 = Close Reference(reference=w283, error in (no error)=w282) -> ()  [unwired: 1 out]
      n76 = Close Reference(reference=w276, error in (no error)=w277) -> ()  [unwired: 1 out]
      n77 = Close Reference(reference=w272, error in (no error)=w275) -> ()  [unwired: 1 out]
      n78 = Close Reference(reference=w271, error in (no error)=w268) -> ()  [unwired: 1 out]
      n79 = Close Reference(reference=w264, error in (no error)=w267) -> ()  [unwired: 1 out]
      n80 = Close Reference(reference=w260, error in (no error)=w261) -> ()  [unwired: 1 out]
      n81 = Close Reference(reference=w256, error in (no error)=w257) -> ()  [unwired: 1 out]
      n82 = Close Reference(reference=w252, error in (no error)=w253) -> ()  [unwired: 1 out]
      n83 = Unbundle By Name(w4) -> ("Motion Module.HomeScratch"=w222:refnum<vi>)
      n84 = Unbundle By Name(w4) -> ("Motion Module.HomeRot"=w225:refnum<vi>)
      n85 = Unbundle By Name(w4) -> ("Motion Module.HomeScratch 2"=w229:refnum<vi>)
      n86 = Unbundle By Name(w4) -> ("Motion Module.Motion Direction:  3"=w234:refnum<vi>)
      n87 = Unbundle By Name(w4) -> ("Motion Module.Motion Mode:"=w237:refnum<vi>)
      n88 = Unbundle By Name(w4) -> ("Motion Module.Rotary Module Selection"=w241:refnum<vi>)
      n89 = Unbundle By Name(w4) -> ("Motion Module.Wear Track Diameter (mm)"=w245:refnum<vi>)
      n90 = Unbundle By Name(w4) -> ("Motion Module.Set WTD"=w249:refnum<vi>)
      n91 = Unbundle By Name(w4) -> ("Motion Module.Motion type:"=w218:refnum<vi>)
      n92 = Unbundle By Name(w4) -> ("Motion Module.Scartch Offset"=w215:refnum<vi>)
      n93 = Unbundle By Name(w4) -> ("Motion Module.Enter Scratch Speed (mm/s):"=w210:refnum<vi>)
      n94 = Unbundle By Name(w4) -> ("Motion Module.Enter Scratch length (mm):"=w206:refnum<vi>)
      n95 = Unbundle By Name(w4) -> ("Motion Module.SwaySpeed Set"=w202:refnum<vi>)
      n96 = Unbundle By Name(w4) -> ("Motion Module.Scratch Mode"=w151:refnum<vi>)
      n97 = Unbundle By Name(w4) -> ("Motion Module.HomeScratch"=w146:refnum<vi>)
      n98 = Unbundle By Name(w4) -> ("Motion Module.No of Scratch"=w66:refnum<vi>)
      n99 = Unbundle By Name(w4) -> ("Motion Module.HomeRot"=w143:refnum<vi>)
      n100 = property class="DigNum (strict)"(reference=w66, "Visible"=FALSE) -> (reference out=w67:refnum<vi>, error out=w65:errorcluster)  [unwired: 1 in]
      n101 = property class="Bool (strict)"(reference=w143, "Visible"=FALSE ("Value")) -> (reference out=w141:refnum<vi>, error out=w144:errorcluster)  [unwired: 1 in]
      n102 = property class="Bool (strict)"(reference=w222, "Value"=FALSE) -> (reference out=w220:refnum<vi>, error out=w221:errorcluster)  [unwired: 1 in]
      n103 = property class="Bool (strict)"(reference=w225, "Value"=FALSE) -> (reference out=w227:refnum<vi>, error out=w226:errorcluster)  [unwired: 1 in]
      n104 = property class="Bool (strict)"(reference=w229, "Visible"=FALSE ("Value")) -> (reference out=w231:refnum<vi>, error out=w228:errorcluster)  [unwired: 1 in]
      n105 = property class="Ring (strict)"(reference=w234, "Visible"=FALSE ("Value")) -> (reference out=w232:refnum<vi>, error out=w235:errorcluster)  [unwired: 1 in]
      n106 = property class="Ring (strict)"(reference=w237, "Visible"=FALSE ("Value")) -> (reference out=w239:refnum<vi>, error out=w236:errorcluster)  [unwired: 1 in]
      n107 = property class="TabCtl (strict)"(reference=w241, "Visible"=FALSE ("Value")) -> (reference out=w243:refnum<vi>, error out=w242:errorcluster)  [unwired: 1 in]
      n108 = property class="DigNum (strict)"(reference=w245, "Visible"=FALSE ("Value")) -> (reference out=w247:refnum<vi>, error out=w246:errorcluster)  [unwired: 1 in]
      n109 = property class="Bool (strict)"(reference=w249, "Visible"=FALSE ("Value")) -> (reference out=w251:refnum<vi>, error out=w250:errorcluster)  [unwired: 1 in]
      n110 = property class="Ring (strict)"(reference=w218, "Visible"=FALSE ("Value")) -> (reference out=w213:refnum<vi>, error out=w217:errorcluster)  [unwired: 1 in]
      n111 = property class="DigNum (strict)"(reference=w215, "Visible"=FALSE ("Value")) -> (reference out=w212:refnum<vi>, error out=w214:errorcluster)  [unwired: 1 in]
      n112 = property class="DigNum (strict)"(reference=w210, "Visible"=FALSE ("Value")) -> (reference out=w208:refnum<vi>, error out=w209:errorcluster)  [unwired: 1 in]
      n113 = property class="DigNum (strict)"(reference=w206, "Visible"=FALSE ("Value")) -> (reference out=w204:refnum<vi>, error out=w205:errorcluster)  [unwired: 1 in]
      n114 = property class="Bool (strict)"(reference=w202, "Visible"=FALSE ("Value")) -> (reference out=w200:refnum<vi>, error out=w201:errorcluster)  [unwired: 1 in]
      n115 = property class="Ring (strict)"(reference=w151, "Visible"=FALSE ("Value")) -> (reference out=w149:refnum<vi>, error out=w152:errorcluster)  [unwired: 1 in]
      n116 = property class="Bool (strict)"(reference=w146, "Visible"=FALSE ("Value")) -> (reference out=w148:refnum<vi>, error out=w145:errorcluster)  [unwired: 1 in]
      n117 = Close Reference(reference=w67, error in (no error)=w65) -> ()  [unwired: 1 out]
      n118 = Close Reference(reference=w141, error in (no error)=w144) -> ()  [unwired: 1 out]
      n119 = Close Reference(reference=w220, error in (no error)=w221) -> ()  [unwired: 1 out]
      n120 = Close Reference(reference=w227, error in (no error)=w226) -> ()  [unwired: 1 out]
      n121 = Close Reference(reference=w231, error in (no error)=w228) -> ()  [unwired: 1 out]
      n122 = Close Reference(reference=w232, error in (no error)=w235) -> ()  [unwired: 1 out]
      n123 = Close Reference(reference=w239, error in (no error)=w236) -> ()  [unwired: 1 out]
      n124 = Close Reference(reference=w243, error in (no error)=w242) -> ()  [unwired: 1 out]
      n125 = Close Reference(reference=w247, error in (no error)=w246) -> ()  [unwired: 1 out]
      n126 = Close Reference(reference=w251, error in (no error)=w250) -> ()  [unwired: 1 out]
      n127 = Close Reference(reference=w213, error in (no error)=w217) -> ()  [unwired: 1 out]
      n128 = Close Reference(reference=w212, error in (no error)=w214) -> ()  [unwired: 1 out]
      n129 = Close Reference(reference=w208, error in (no error)=w209) -> ()  [unwired: 1 out]
      n130 = Close Reference(reference=w204, error in (no error)=w205) -> ()  [unwired: 1 out]
      n131 = Close Reference(reference=w200, error in (no error)=w201) -> ()  [unwired: 1 out]
      n132 = Close Reference(reference=w149, error in (no error)=w152) -> ()  [unwired: 1 out]
      n133 = Close Reference(reference=w148, error in (no error)=w145) -> ()  [unwired: 1 out]
      n134 = Unbundle By Name(w4) -> ("Environmental control.High Temp"=w170:refnum<vi>)
      n135 = Unbundle By Name(w4) -> ("Environmental control.Low Temp"=w173:refnum<vi>)
      n136 = Unbundle By Name(w4) -> ("Environmental control.Humidity"=w177:refnum<vi>)
      n137 = Unbundle By Name(w4) -> ("Environmental control.Enter the Stage \nTemperature (°C):"=w182:refnum<vi>)
      n138 = Unbundle By Name(w4) -> ("Environmental control.Enter the Temperature (°C):"=w185:refnum<vi>)
      n139 = Unbundle By Name(w4) -> ("Environmental control.Enter the Humidity (%Rh):"=w189:refnum<vi>)
      n140 = Unbundle By Name(w4) -> ("Environmental control.Stage Temperature"=w193:refnum<vi>)
      n141 = Unbundle By Name(w4) -> ("Environmental control.Sample Temperature"=w197:refnum<vi>)
      n142 = Unbundle By Name(w4) -> ("Main Screen.zNL 2"=w168:refnum<vi>)
      n143 = Unbundle By Name(w4) -> ("Main Screen.Load En"=w164:refnum<vi>)
      n144 = Unbundle By Name(w4) -> ("Main Screen.CZ FF"=w158:refnum<vi>)
      n145 = Unbundle By Name(w4) -> ("Main Screen.zFF"=w155:refnum<vi>)
      n146 = property class="DigNum (strict)"(reference=w182, "Visible"=FALSE ("Value")) -> (reference out=w180:refnum<vi>, error out=w183:errorcluster)  [unwired: 1 in]
      n147 = property class="DigNum (strict)"(reference=w185, "Visible"=FALSE ("Value")) -> (reference out=w187:refnum<vi>, error out=w184:errorcluster)  [unwired: 1 in]
      n148 = property class="DigNum (strict)"(reference=w189, "Visible"=FALSE ("Value")) -> (reference out=w191:refnum<vi>, error out=w190:errorcluster)  [unwired: 1 in]
      n149 = property class="Bool (strict)"(reference=w170, "Value"=FALSE) -> (reference out=w140:refnum<vi>, error out=w169:errorcluster)  [unwired: 1 in]
      n150 = property class="Bool (strict)"(reference=w173, "Value"=FALSE) -> (reference out=w175:refnum<vi>, error out=w174:errorcluster)  [unwired: 1 in]
      n151 = property class="Bool (strict)"(reference=w177, "Value"=FALSE) -> (reference out=w179:refnum<vi>, error out=w176:errorcluster)  [unwired: 1 in]
      n152 = property class="Bool (strict)"(reference=w168, "DisabledEnum"=T2."Enabled" ("Disabled")) -> (reference out=w166:refnum<vi>, error out=w167:errorcluster)  [unwired: 1 in]
      n153 = property class="Bool (strict)"(reference=w164, "DisabledEnum"=T2."Enabled" ("Disabled")) -> (reference out=w162:refnum<vi>, error out=w163:errorcluster)  [unwired: 1 in]
      n154 = property class="Bool (strict)"(reference=w158, "DisabledEnum"=T2."Enabled" ("Disabled")) -> (reference out=w157:refnum<vi>, error out=w159:errorcluster)  [unwired: 1 in]
      n155 = property class="Bool (strict)"(reference=w155, "DisabledEnum"=T2."Enabled" ("Disabled")) -> (reference out=w156:refnum<vi>, error out=w154:errorcluster)  [unwired: 1 in]
      n156 = property class="Arr (strict)"(reference=w193, "Visible"=FALSE ("Value")) -> (reference out=w195:refnum<vi>, error out=w194:errorcluster)  [unwired: 1 in]
      n157 = property class="Arr (strict)"(reference=w197, "Visible"=FALSE ("Value")) -> (reference out=w199:refnum<vi>, error out=w198:errorcluster)  [unwired: 1 in]
      n158 = Close Reference(reference=w140, error in (no error)=w169) -> ()  [unwired: 1 out]
      n159 = Close Reference(reference=w175, error in (no error)=w174) -> ()  [unwired: 1 out]
      n160 = Close Reference(reference=w179, error in (no error)=w176) -> ()  [unwired: 1 out]
      n161 = Close Reference(reference=w180, error in (no error)=w183) -> ()  [unwired: 1 out]
      n162 = Close Reference(reference=w187, error in (no error)=w184) -> ()  [unwired: 1 out]
      n163 = Close Reference(reference=w191, error in (no error)=w190) -> ()  [unwired: 1 out]
      n164 = Close Reference(reference=w195, error in (no error)=w194) -> ()  [unwired: 1 out]
      n165 = Close Reference(reference=w199, error in (no error)=w198) -> ()  [unwired: 1 out]
      n166 = Close Reference(reference=w166, error in (no error)=w167) -> ()  [unwired: 1 out]
      n167 = Close Reference(reference=w162, error in (no error)=w163) -> ()  [unwired: 1 out]
      n168 = Close Reference(reference=w157, error in (no error)=w159) -> ()  [unwired: 1 out]
      n169 = Close Reference(reference=w156, error in (no error)=w154) -> ()  [unwired: 1 out]
      n170 = Unbundle By Name(w4) -> ("Environmental control.Sensors Picked"=w97:refnum<vi>)
      n171 = Unbundle By Name(w4) -> ("Environmental control.Acoustic Emission 3"=w138:refnum<vi>)
      n172 = Unbundle By Name(w4) -> ("Environmental control.ECR"=w134:refnum<vi>)
      n173 = Unbundle By Name(w4) -> ("Environmental control.Temperature (Amb)"=w132:refnum<vi>)
      n174 = Unbundle By Name(w4) -> ("Environmental control.Temperature (Chamber)"=w129:refnum<vi>)
      n175 = Unbundle By Name(w4) -> ("Environmental control.Humidity (Chamber)"=w126:refnum<vi>)
      n176 = Unbundle By Name(w4) -> ("Environmental control.Microphone"=w123:refnum<vi>)
      n177 = Unbundle By Name(w4) -> ("Environmental control.Wear"=w120:refnum<vi>)
      n178 = Unbundle By Name(w4) -> ("Environmental control.Vibration"=w117:refnum<vi>)
      n179 = Unbundle By Name(w4) -> ("Main Screen.Test Trip"=w106:refnum<vi>)
      n180 = Unbundle By Name(w4) -> ("Main Screen.Trip Log"=w102:refnum<vi>)
      n181 = property class="Bool (strict)"(reference=w138, "Value"=FALSE) -> (reference out=w139:refnum<vi>, error out=w137:errorcluster)  [unwired: 1 in]
      n182 = property class="Bool (strict)"(reference=w134, "Value"=FALSE) -> (reference out=w136:refnum<vi>, error out=w135:errorcluster)  [unwired: 1 in]
      n183 = property class="Bool (strict)"(reference=w132, "Value"=FALSE) -> (reference out=w131:refnum<vi>, error out=w133:errorcluster)  [unwired: 1 in]
      n184 = property class="Bool (strict)"(reference=w129, "Value"=FALSE) -> (reference out=w130:refnum<vi>, error out=w128:errorcluster)  [unwired: 1 in]
      n185 = property class="Bool (strict)"(reference=w126, "Value"=FALSE) -> (reference out=w125:refnum<vi>, error out=w127:errorcluster)  [unwired: 1 in]
      n186 = property class="Bool (strict)"(reference=w123, "Value"=FALSE) -> (reference out=w124:refnum<vi>, error out=w122:errorcluster)  [unwired: 1 in]
      n187 = property class="Bool (strict)"(reference=w120, "Value"=FALSE) -> (reference out=w119:refnum<vi>, error out=w121:errorcluster)  [unwired: 1 in]
      n188 = property class="Bool (strict)"(reference=w117, "Value"=FALSE) -> (reference out=w118:refnum<vi>, error out=w116:errorcluster)  [unwired: 1 in]
      n189 = property class="Bool (strict)"(reference=w106, "Value"=FALSE) -> (reference out=w107:refnum<vi>, error out=w105:errorcluster)  [unwired: 1 in]
      n190 = property class="Str"(reference=w102, "Value"="") -> (reference out=w101:refnum<vi>, error out=w103:errorcluster)  [unwired: 1 in]
      n191 = property class="Str"(reference=w97, "Value"="") -> (reference out=w98:refnum<vi>, error out=w96:errorcluster)  [unwired: 1 in]
      n192 = Close Reference(reference=w139, error in (no error)=w137) -> ()  [unwired: 1 out]
      n193 = Close Reference(reference=w136, error in (no error)=w135) -> ()  [unwired: 1 out]
      n194 = Close Reference(reference=w131, error in (no error)=w133) -> ()  [unwired: 1 out]
      n195 = Close Reference(reference=w130, error in (no error)=w128) -> ()  [unwired: 1 out]
      n196 = Close Reference(reference=w125, error in (no error)=w127) -> ()  [unwired: 1 out]
      n197 = Close Reference(reference=w124, error in (no error)=w122) -> ()  [unwired: 1 out]
      n198 = Close Reference(reference=w119, error in (no error)=w121) -> ()  [unwired: 1 out]
      n199 = Close Reference(reference=w118, error in (no error)=w116) -> ()  [unwired: 1 out]
      n200 = Close Reference(reference=w107, error in (no error)=w105) -> ()  [unwired: 1 out]
      n201 = Close Reference(reference=w101, error in (no error)=w103) -> ()  [unwired: 1 out]
      n202 = Close Reference(reference=w98, error in (no error)=w96) -> ()  [unwired: 1 out]
      n203 = Unbundle By Name(w4) -> ("About Screen.Heave and Surge COM Port:"=w94:refnum<vi>)
      n204 = Unbundle By Name(w4) -> ("About Screen.Sway COM Port:"=w91:refnum<vi>)
      n205 = Unbundle By Name(w4) -> ("About Screen.Temp Modbus:"=w88:refnum<vi>)
      n206 = Unbundle By Name(w4) -> ("About Screen.Humidity Port:"=w87:refnum<vi>)
      n207 = Unbundle By Name(w4) -> ("About Screen.Ramp Port:"=w73:refnum<vi>)
      n208 = Unbundle By Name(w4) -> ("About Screen.Password"=w82:refnum<vi>)
      n209 = Unbundle By Name(w4) -> ("About Screen.ECR Port:"=w72:refnum<vi>)
      n210 = property class="VISAName"(reference=w94, "DisabledEnum"=T2."Disabled and Grayed Out" ("Disabled")) -> (reference out=w95:refnum<vi>, error out=w93:errorcluster)  [unwired: 1 in]
      n211 = property class="VISAName"(reference=w91, "DisabledEnum"=T2."Disabled and Grayed Out" ("Disabled")) -> (reference out=w92:refnum<vi>, error out=w90:errorcluster)  [unwired: 1 in]
      n212 = property class="VISAName"(reference=w88, "DisabledEnum"=T2."Disabled and Grayed Out" ("Disabled")) -> (reference out=w76:refnum<vi>, error out=w89:errorcluster)  [unwired: 1 in]
      n213 = property class="VISAName"(reference=w87, "DisabledEnum"=T2."Disabled and Grayed Out" ("Disabled")) -> (reference out=w85:refnum<vi>, error out=w86:errorcluster)  [unwired: 1 in]
      n214 = property class="VISAName"(reference=w73, "DisabledEnum"=T2."Disabled and Grayed Out" ("Disabled")) -> (reference out=w68:refnum<vi>, error out=w74:errorcluster)  [unwired: 1 in]
      n215 = property class="VISAName"(reference=w72, "DisabledEnum"=T2."Disabled and Grayed Out" ("Disabled")) -> (reference out=w69:refnum<vi>, error out=w71:errorcluster)  [unwired: 1 in]
      n216 = property class="Str"(reference=w82, "Visible"=FALSE) -> (reference out=w84:refnum<vi>, error out=w83:errorcluster)  [unwired: 1 in]
      n217 = Close Reference(reference=w95, error in (no error)=w93) -> ()  [unwired: 1 out]
      n218 = Close Reference(reference=w92, error in (no error)=w90) -> ()  [unwired: 1 out]
      n219 = Close Reference(reference=w76, error in (no error)=w89) -> ()  [unwired: 1 out]
      n220 = Close Reference(reference=w85, error in (no error)=w86) -> ()  [unwired: 1 out]
      n221 = Close Reference(reference=w84, error in (no error)=w83) -> ()  [unwired: 1 out]
      n222 = Close Reference(reference=w68, error in (no error)=w74) -> ()  [unwired: 1 out]
      n223 = Close Reference(reference=w69, error in (no error)=w71) -> ()  [unwired: 1 out]
      n224 = Unbundle By Name(w4) -> ("Traction reciepe.SRR Sweep Range (%) Stribeck"=w46:refnum<vi>)
      n225 = Unbundle By Name(w4) -> ("Traction reciepe.Traction Receipe"=w49:refnum<vi>)
      n226 = Unbundle By Name(w4) -> ("Traction reciepe.Total Execution Time"=w52:refnum<vi>)
      n227 = Unbundle By Name(w4) -> ("Traction reciepe.Total Steps"=w44:refnum<vi>)
      n228 = Unbundle By Name(w4) -> ("Traction reciepe.Duration / Step (s)  Stribeck"=w41:refnum<vi>)
      n229 = Unbundle By Name(w4) -> ("Traction reciepe.STRIBECK Fixed SRR List (%)"=w38:refnum<vi>)
      n230 = Unbundle By Name(w4) -> ("Traction reciepe.Duration / Step (s) Traction"=w61:refnum<vi>)
      n231 = Unbundle By Name(w4) -> ("Traction reciepe.SRR Sweep Range (%) traction"=w25:refnum<vi>)
      n232 = Unbundle By Name(w4) -> ("Traction reciepe.Rolling Speed (mm/s)"=w22:refnum<vi>)
      n233 = Unbundle By Name(w4) -> ("Traction reciepe.Temperature Stages (°C)"=w19:refnum<vi>)
      n234 = Unbundle By Name(w4) -> ("Traction reciepe.Ball Load (N)"=w27:refnum<vi>)
      n235 = Unbundle By Name(w4) -> ("Traction reciepe.Lubricant Name"=w30:refnum<vi>)
      n236 = Unbundle By Name(w4) -> ("Traction reciepe.Profile File Name"=w33:refnum<vi>)
      n237 = property class="Str"(reference=w46, "Visible"=FALSE) -> (reference out=w47:refnum<vi>, error out=w45:errorcluster)  [unwired: 1 in]
      n238 = property class="MCListbox (strict)"(reference=w49, "Visible"=FALSE) -> (reference out=w48:refnum<vi>, error out=w50:errorcluster)  [unwired: 1 in]
      n239 = property class="DigNum (strict)"(reference=w52, "Visible"=FALSE) -> (reference out=w53:refnum<vi>, error out=w51:errorcluster)  [unwired: 1 in]
      n240 = property class="DigNum (strict)"(reference=w44, "Visible"=FALSE) -> (reference out=w39:refnum<vi>, error out=w43:errorcluster)  [unwired: 1 in]
      n241 = property class="DigNum (strict)"(reference=w41, "Visible"=FALSE) -> (reference out=w40:refnum<vi>, error out=w42:errorcluster)  [unwired: 1 in]
      n242 = property class="Str"(reference=w38, "Visible"=FALSE) -> (reference out=w36:refnum<vi>, error out=w37:errorcluster)  [unwired: 1 in]
      n243 = property class="DigNum (strict)"(reference=w61, "Visible"=FALSE) -> (reference out=w63:refnum<vi>, error out=w62:errorcluster)  [unwired: 1 in]
      n244 = property class="Str"(reference=w25, "Visible"=FALSE) -> (reference out=w24:refnum<vi>, error out=w26:errorcluster)  [unwired: 1 in]
      n245 = property class="DigNum (strict)"(reference=w22, "Visible"=FALSE) -> (reference out=w23:refnum<vi>, error out=w21:errorcluster)  [unwired: 1 in]
      n246 = property class="Str"(reference=w19, "Visible"=FALSE) -> (reference out=w18:refnum<vi>, error out=w20:errorcluster)  [unwired: 1 in]
      n247 = property class="Str"(reference=w27, "Visible"=FALSE) -> (reference out=w32:refnum<vi>, error out=w28:errorcluster)  [unwired: 1 in]
      n248 = property class="Str"(reference=w30, "Visible"=FALSE) -> (reference out=w31:refnum<vi>, error out=w29:errorcluster)  [unwired: 1 in]
      n249 = property class="Str"(reference=w33, "Visible"=FALSE) -> (reference out=w35:refnum<vi>, error out=w34:errorcluster)  [unwired: 1 in]
      n250 = Close Reference(reference=w47, error in (no error)=w45) -> ()  [unwired: 1 out]
      n251 = Close Reference(reference=w48, error in (no error)=w50) -> ()  [unwired: 1 out]
      n252 = Close Reference(reference=w53, error in (no error)=w51) -> ()  [unwired: 1 out]
      n253 = Close Reference(reference=w39, error in (no error)=w43) -> ()  [unwired: 1 out]
      n254 = Close Reference(reference=w40, error in (no error)=w42) -> ()  [unwired: 1 out]
      n255 = Close Reference(reference=w36, error in (no error)=w37) -> ()  [unwired: 1 out]
      n256 = Close Reference(reference=w63, error in (no error)=w62) -> ()  [unwired: 1 out]
      n257 = Close Reference(reference=w24, error in (no error)=w26) -> ()  [unwired: 1 out]
      n258 = Close Reference(reference=w23, error in (no error)=w21) -> ()  [unwired: 1 out]
      n259 = Close Reference(reference=w18, error in (no error)=w20) -> ()  [unwired: 1 out]
      n260 = Close Reference(reference=w32, error in (no error)=w28) -> ()  [unwired: 1 out]
      n261 = Close Reference(reference=w31, error in (no error)=w29) -> ()  [unwired: 1 out]
      n262 = Close Reference(reference=w35, error in (no error)=w34) -> ()  [unwired: 1 out]
      n263 = Unbundle By Name(w4) -> ("Environmental control.Acoustic Emission 3"=w9:refnum<vi>)
      n264 = Unbundle By Name(w4) -> ("Acquostic.Gains"=w8:refnum<vi>)
      n265 = property class="RadioBtnsControl (strict)"(reference=w8, "Visible"=FALSE) -> (reference out=w3:refnum<vi>, error out=w7:errorcluster)  [unwired: 1 in]
      n266 = property class="Bool (strict)"(reference=w9, "Value"=FALSE ("Visible")) -> (reference out=w11:refnum<vi>, error out=w10:errorcluster)  [unwired: 1 in]
      n267 = Close Reference(reference=w3, error in (no error)=w7) -> ()  [unwired: 1 out]
      n268 = Close Reference(reference=w11, error in (no error)=w10) -> ()  [unwired: 1 out]
    }
    frame Error {
    }
  }
